vi "Logging Message Loop.vi"(8 "error in (no error)":errorcluster, 10 "DataQueuesAndNotifier":T1, 11 "Message Queues":T2) -> (0 "error out":errorcluster)   [LabVIEW 2019, in "Logging.lvlib"]
doc: "The message loop subVI to handle messages pertaining to logging data."
uses:
  Logging.lvlib
  support/Message Queue/All Message Queues.ctl
  support/Message Queue/Message Cluster.ctl
  Acquisition/DataQueuesAndNotifier.ctl
  Logging State.ctl
  Settings/Settings.ctl
  HardwareAdapter/Support/Hardware Configuration.ctl
  HardwareAdapter/Support/Camera Configuration.ctl
  <vilib>/userdefined/High Color/IMAQdx.ctl
  Logging Configuration.ctl
  controls/UI Configuration.ctl
  controls/CallBack Refs.ctl
  support/Message Queue/Enqueue Message (Single).vi
  <vilib>/Utility/error.llb/Error Cluster From Error Code.vi
  D:/SDK/PMQI-LabViewSamples/Examples/Dependencies/PVCamNET.dll
  E:/DevHardSoftware/MMicroscopy/HardwareAdapter/Lasers/Dependencies/Oxxius_Boxx.dll
  HardwareAdapter/Lasers/Dependencies/Oxxius_Boxx.dll
  <vilib>/ErrorRing/Error Ring.xnode
  support/Message Queue/Message Queue.lvlib
  Settings/Settings.lvlib
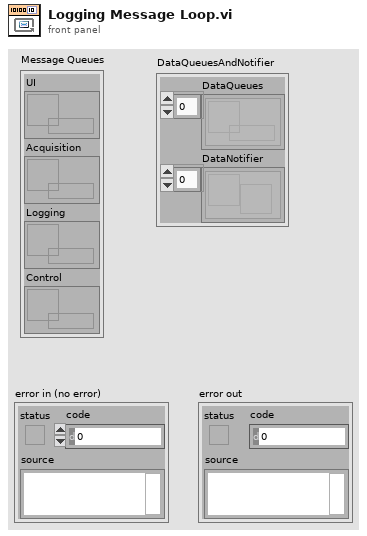
[diagram p1: front panel]
types:
  T1 = typedef "DataQueuesAndNotifier.ctl" = cluster{"DataQueues":refnum<queue>[], "DataNotifier":refnum<notifier>[]}
  T2 = typedef "Message Queue.lvlib/All Message Queues.ctl" = cluster{"UI":refnum<queue>, "Acquisition":refnum<queue>, "Logging":refnum<queue>, "Control":refnum<queue>}
  T3 = typedef "Logging.lvlib/Logging State.ctl" = enum16{"Idle", "Logging"}
  T4 = typedef "Settings.lvlib/Settings.ctl" = cluster{"Hardware Configuration":T5, "Logging Configuration":T8, "HardWare Status":cluster{"CameraAndStages":T9, "Lasers":cluster{"IsConnected":cluster{"405":bool, "488":bool, "532":bool, "561":bool, "647":bool, "785":bool}, "IsOpened":cluster{"405":bool, "488":bool, "532":bool, "561":bool, "647":bool, "785":bool}}}, "CallBack Ref":T10}
  T5 = typedef "Hardware Configuration.ctl" = cluster{"Camera Configuration":T6, "SimpleCamera Configuration":cluster{"Resource":cluster{"Session Out":T7}}, "Stages Configuration":cluster{"Resource":cluster{"NanoStage Ref":i32, "MicroStage Ref":i32, "TirfLock Ref":i32}, "SettingValues":cluster{"NanoState":cluster{"Time":dbl, "X":dbl, "Y":dbl, "Z":dbl}, "MicroState":cluster{"Time 2":dbl, "Z":dbl}, "TirfLock":cluster{"Time":dbl, "X":dbl, "Y":dbl, "Sum":dbl, "Calbrate":dbl, "LockedTarget":dbl, "Kp":dbl, "Ki":dbl, "Avg":dbl}}}, "Lasers Configuration":cluster{"SettingValues":cluster{"405 Power":sgl, "488 Power":sgl, "532 Power":sgl, "561 Power":sgl, "647 Power":sgl, "785 Power":sgl}, "Resource":cluster{"Library Ref":refnum<k24>, "Lasers Ref":cluster{"405 Ref":refnum<k24>, "488 Ref":refnum<k24>, "532 Ref":refnum<k24>, "561 Ref":refnum<k24>, "647 Ref":refnum<k24>, "785 Ref":refnum<k24>}}}}
  T6 = typedef "Camera Configuration.ctl" = cluster{"Resource":cluster{"CameraRef":refnum<k24>, "LibraryRef":refnum<k24>}, "Setting":cluster{"Expouse":dbl, "Frames":dbl, "FrameRate":dbl}}
  T7 = typedef "IMAQdx.ctl" = refnum<k21>
  T8 = typedef "Logging.lvlib/Logging Configuration.ctl" = cluster{"Log File Base Path":path, "FilePrefix":string, "TiffFileFullPath":path, "HardWareInfoFileFullPath":path, "NoteFileFullPath":path}
  T9 = typedef "UI Configuration.ctl" = cluster{"Camera":bool, "NanoStage":bool, "MicroStage":bool, "TIRFLock":bool}
  T10 = typedef "CallBack Refs.ctl" = cluster{"event callback refnum":refnum<k27>, "event callback refnum 2":refnum<k27>, "event callback refnum 3":refnum<k27>, "event callback refnum 4":refnum<k27>}
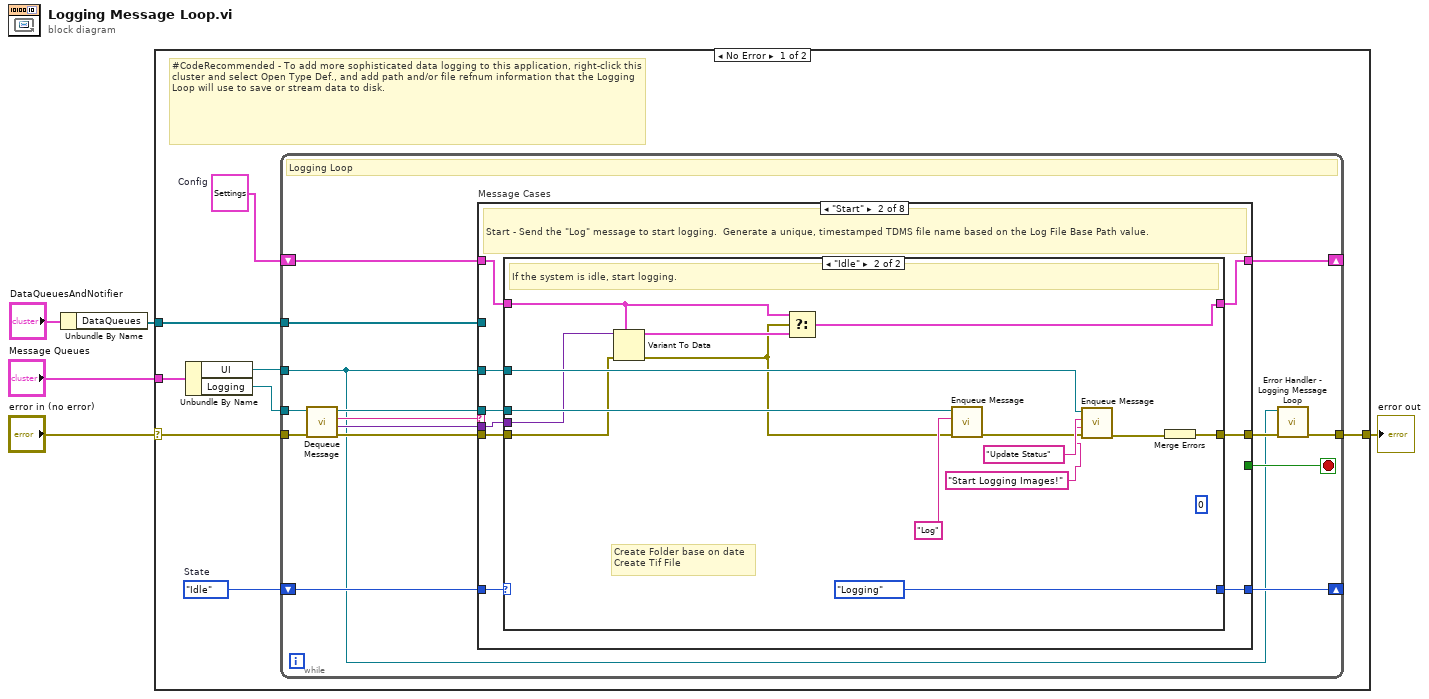
[diagram p0: block diagram]
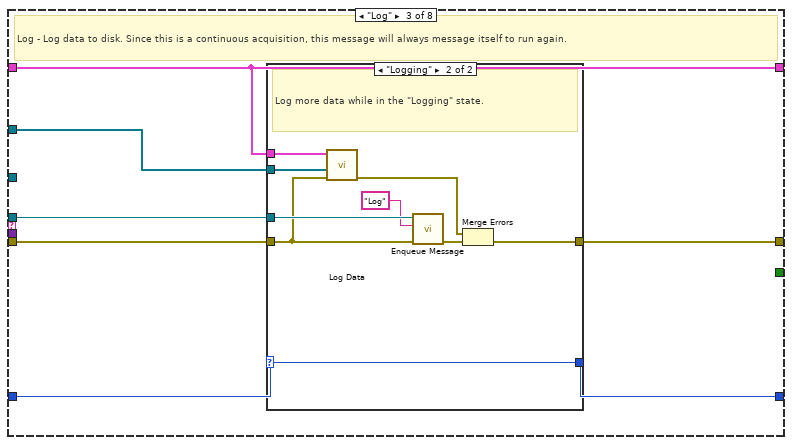
[diagram p4: hidden frame]
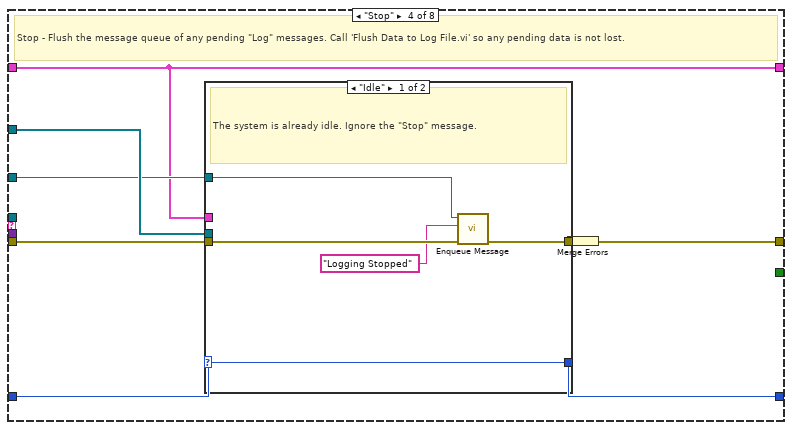
[diagram p6: hidden frame]
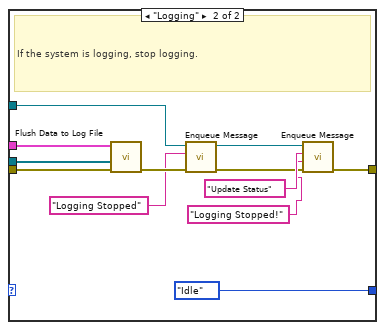
[diagram p7: hidden frame]
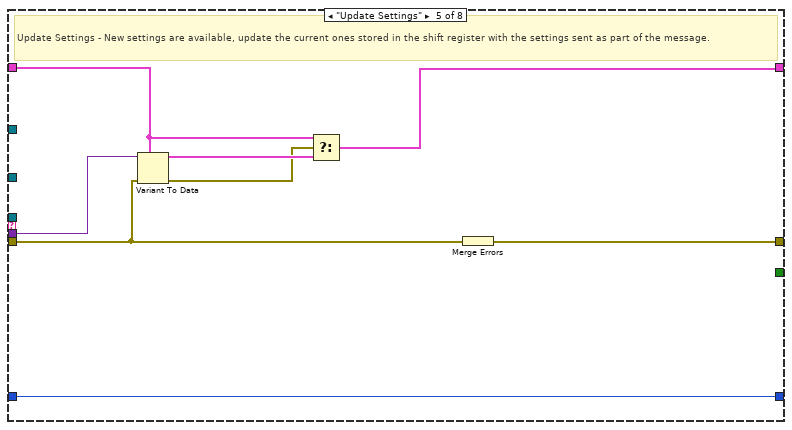
[diagram p8: hidden frame]
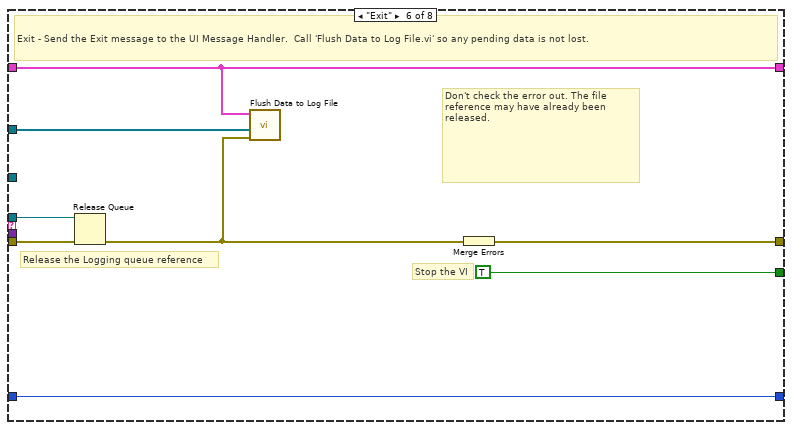
[diagram p9: hidden frame]
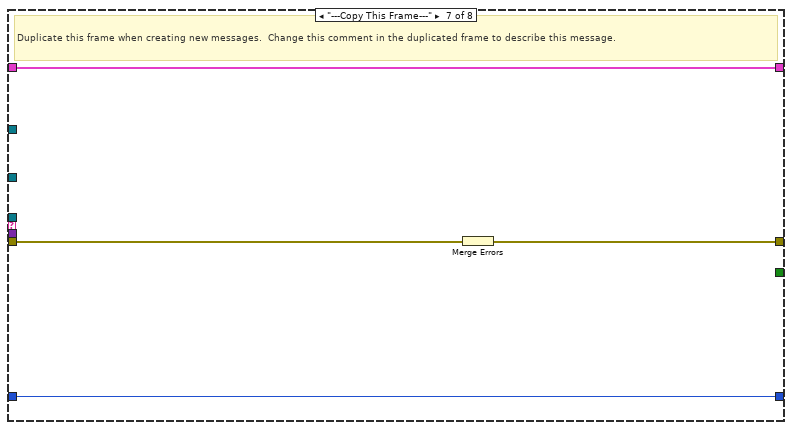
[diagram p10: hidden frame]
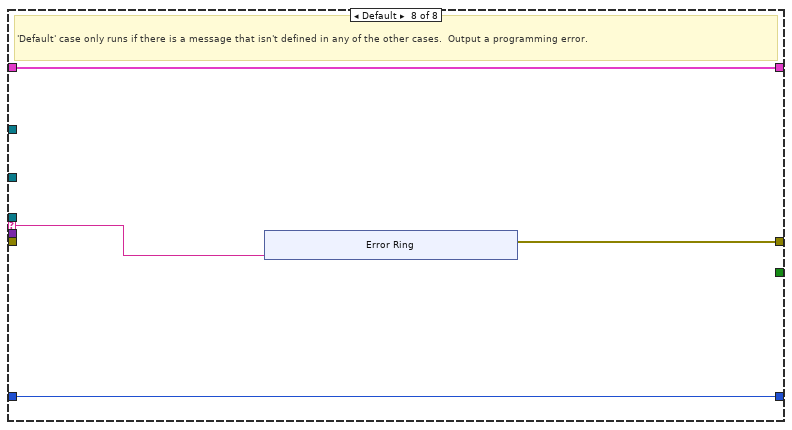
[diagram p11: hidden frame]
diagram:
  n1 = Unbundle By Name("DataQueuesAndNotifier") -> ("DataQueues"=w1:refnum<queue>[])
  n2 = case shown="No Error" "error in (no error)" {
    selector: "error in (no error)" -> [w10 w133]
    tunnel: "Message Queues" -> [w13 _]
    tunnel: [w11 w133] -> w4
    tunnel: w1 -> [w9 _]
    frame No Error {
      w6 = T4 {"Hardware Configuration"={"Camera Configuration"={"Resource"={"CameraRef"=refnum, "LibraryRef"=refnum}, "Setting"={"Expouse"=0.0, "Frames"=0.0, "FrameRate"=0.0}}, "SimpleCamera Configuration"={"Resource"={"Session Out"=""}}, "Stages Configuration"={"Resource"={"NanoStage Ref"=0, "MicroStage Ref"=0, "TirfLock Ref"=0}, "SettingValues"={"NanoState"={"Time"=0.0, "X"=0.0, "Y"=0.0, "Z"=0.0}, "MicroState"={"Time 2"=0.0, "Z"=0.0}, "TirfLock"={"Time"=0.0, "X"=0.0, "Y"=0.0, "Sum"=0.0, "Calbrate"=0.0, "LockedTarget"=0.0, "Kp"=0.0, "Ki"=0.0, "Avg"=0.0}}}, "Lasers Configuration"={"SettingValues"={"405 Power"=0.0, "488 Power"=0.0, "532 Power"=0.0, "561 Power"=0.0, "647 Power"=0.0, "785 Power"=0.0}, "Resource"={"Library Ref"=refnum, "Lasers Ref"={"405 Ref"=refnum, "488 Ref"=refnum, "532 Ref"=refnum, "561 Ref"=refnum, "647 Ref"=refnum, "785 Ref"=refnum}}}}, "Logging Configuration"={"Log File Base Path"=path "", "FilePrefix"="", "TiffFileFullPath"=path "", "HardWareInfoFileFullPath"=path "", "NoteFileFullPath"=path ""}, "HardWare Status"={"CameraAndStages"={"Camera"=FALSE, "NanoStage"=FALSE, "MicroStage"=FALSE, "TIRFLock"=FALSE}, "Lasers"={"IsConnected"={"405"=FALSE, "488"=FALSE, "532"=FALSE, "561"=FALSE, "647"=FALSE, "785"=FALSE}, "IsOpened"={"405"=FALSE, "488"=FALSE, "532"=FALSE, "561"=FALSE, "647"=FALSE, "785"=FALSE}}}, "CallBack Ref"={"event callback refnum"=refnum, "event callback refnum 2"=refnum, "event callback refnum 3"=refnum, "event callback refnum 4"=refnum}}  # Config
      w7 = Logging_State."Idle"  # State
      # "#CodeRecommended - To add more sophisticated data logging to this application, right-click this cluster and select Open Type Def., and add path and/or file refnum information that the Logging Loop will use to save or stream data to disk."
      n3 = Unbundle By Name(w13) -> ("UI"=w8:refnum<queue>, "Logging"=w12:refnum<queue>)
      n4 = while {
        tunnel: w12 -> [w20]
        shift-right: [w27] -> _
        shift-left: w6 -> [w28]
        tunnel: w8 -> [w14]
        tunnel: w9 -> [w19]
        shift-right: [w17] -> _
        shift-left: w7 -> [w18]
        tunnel: w10 -> [w25]
        tunnel: [w16] -> w11
        stop <- w26 stop-if-true
        # "Logging Loop"
        n5 = call "Dequeue Message.vi"("error in (no error)"=w25, "Message Queue"=w20) -> ("error out"=w24:errorcluster, "Message Data"=w22:variant, "Message"=w23:string, "dup Message Queue"=w21:refnum<queue>)  [unwired: 6 in]
        n6 = case "Message Cases" shown="\"Start\"" w23 {
          selector: w23 -> [_ _ _ _ _ _ _ w122]
          tunnel: w21 -> [_ w39 w64 _ _ w114 _ _]
          tunnel: w24 -> [w30 w38 w62 w81 w103 w115 w121 _]
          tunnel: [w30 w40 w65 w84 w109 w116 w119 w123] -> w15
          tunnel: w28 -> [w31 w37 w61 w77 w107 w112 w120 w125]
          tunnel: [w31 w36 w61 w77 w104 w112 w120 w125] -> w27
          tunnel: [_ _ _ _ _ TRUE _ _] -> w26
          tunnel: w22 -> [_ w32 _ _ w108 _ _ _]
          tunnel: w14 -> [_ w33 _ w78 _ _ _ _]
          tunnel: w19 -> [_ _ w63 w82 _ w110 _ _]
          tunnel: w18 -> [w29 w35 w60 w80 w102 w111 w118 w124]
          tunnel: [w29 w34 w59 w79 w102 w111 w118 w124] -> w17
          frame "Initialize" {
            # "Initialize - gets called when first launched. Currently a no-op."
          }
          frame "Start" {
            # "Start - Send the \"Log\" message to start logging.  Generate a unique, timestamped TDMS file name based on the Log File Base Path value."
            n7 = case shown="\"Idle\"" w35 {
              selector: w35 -> [w42 _]
              tunnel: [w41 w57] -> w40
              tunnel: w39 -> [_ w56]
              tunnel: w38 -> [w41 w45]
              tunnel: w37 -> [w43 w47]
              tunnel: [w43 w46] -> w36
              tunnel: [w42 Logging_State."Logging" ("State")] -> w34
              tunnel: w33 -> [_ w50]
              tunnel: w32 -> [_ w48]
              frame "Logging" {
                # "The system is already logging. Ignore the \"Start\" message."
              }
              frame "Idle" {
                (unwired) 0 ("CurrentCaptureFrame")
                # "Create Folder base on date\nCreate Tif File"
                # "If the system is idle, start logging."
                n8 = Variant To Data(error in=w45, type=w47, Variant=w48) -> (data=w49:T4, error out=w44:errorcluster)
                n9 = Select(t=w47, s=w44, f=w49) -> (s? t:f=w46:T4)
                n10 = call-poly "Enqueue Message.vi"("error in (no error)"=w44, "Message"="Log", "Message Queue"=w56) -> ("error out"=w52:errorcluster)  [unwired: 7 in, 1 out]
                n11 = call-poly "Enqueue Message.vi"("error in (no error)"=w52, "Message Data"="Start Logging Images!" ("Message"), "Message"="Update Status", "Message Queue"=w50) -> ("error out"=w51:errorcluster)  [unwired: 6 in, 1 out]
                n12 = Merge Errors(w51) -> (w57:errorcluster)
              }
            }
          }
          frame "Log" {
            # "Log - Log data to disk. Since this is a continuous acquisition, this message will always message itself to run again."
            n13 = case shown="\"Logging\"" w60 {
              selector: w60 -> [w67 w70]
              tunnel: [w66 w76] -> w65
              tunnel: w64 -> [_ w74]
              tunnel: w63 -> [_ w68]
              tunnel: w62 -> [w66 w69]
              tunnel: w61 -> [_ w71]
              tunnel: [w67 w70] -> w59
              frame "Idle" {
                # "Ignore \"Log\" messages when the logging is idle."
              }
              frame "Logging" {
                # "Log more data while in the \"Logging\" state."
                n14 = call "Log Data.vi"("error in (no error)"=w69, "DataQueues"=w68, "Config"=w71) -> ("error out"=w73:errorcluster)  [unwired: 8 in]
                n15 = call-poly "Enqueue Message.vi"("error in (no error)"=w69, "Message"="Log", "Message Queue"=w74) -> ("error out"=w75:errorcluster)  [unwired: 7 in, 1 out]
                n16 = Merge Errors(w73, w75) -> (w76:errorcluster)
              }
            }
          }
          frame "Stop" {
            # "Stop - Flush the message queue of any pending \"Log\" messages. Call 'Flush Data to Log File.vi' so any pending data is not lost."
            n17 = case shown="\"Idle\"" w80 {
              selector: w80 -> [w89 _]
              tunnel: [w87 w91] -> w83
              tunnel: w82 -> [_ w95]
              tunnel: w77 -> [_ w100]
              tunnel: w81 -> [w88 w99]
              tunnel: [w89 Logging_State."Idle" ("State")] -> w79
              tunnel: w78 -> [w85 w97]
              frame "Idle" {
                # "The system is already idle. Ignore the \"Stop\" message."
                n18 = call-poly "Enqueue Message.vi"("error in (no error)"=w88, "Message"="Logging Stopped", "Message Queue"=w85) -> ("error out"=w87:errorcluster)  [unwired: 7 in, 1 out]
              }
              frame "Logging" {
                # "If the system is logging, stop logging."
                n19 = call "Flush Data to Log File.vi"("error in (no error)"=w99, "DataQueues"=w95, "Config"=w100) -> ("error out"=w101:errorcluster)  [unwired: 8 in]
                n20 = call-poly "Enqueue Message.vi"("error in (no error)"=w101, "Message"="Logging Stopped", "Message Queue"=w97) -> ("error out"=w92:errorcluster, "dup Message Queue"=w90:refnum<queue>)  [unwired: 7 in]
                n21 = call-poly "Enqueue Message.vi"("error in (no error)"=w92, "Message Data"="Logging Stopped!" ("Message"), "Message"="Update Status", "Message Queue"=w90) -> ("error out"=w91:errorcluster)  [unwired: 6 in, 1 out]
              }
            }
            n22 = Merge Errors(w83) -> (w84:errorcluster)
          }
          frame "Update Settings" {
            # "Update Settings - New settings are available, update the current ones stored in the shift register with the settings sent as part of the message."
            n23 = Variant To Data(error in=w103, type=w107, Variant=w108) -> (data=w106:T4, error out=w105:errorcluster)
            n24 = Select(t=w107, s=w105, f=w106) -> (s? t:f=w104:T4)
            n25 = Merge Errors(w103) -> (w109:errorcluster)
          }
          frame "Exit" {
            # "Don't check the error out. The file reference may have already been released."
            # "Release the Logging queue reference"
            # "Stop the VI"
            # "Exit - Send the Exit message to the UI Message Handler.  Call 'Flush Data to Log File.vi' so any pending data is not lost."
            n26 = Release Queue(queue=w114, error in (no error)=w115) -> (error out=w113:errorcluster)  [unwired: 1 in, 2 out]
            n27 = call "Flush Data to Log File.vi"("error in (no error)"=w113, "DataQueues"=w110, "Config"=w112) -> ()  [unwired: 8 in, 1 out]
            n28 = Merge Errors(w113) -> (w116:errorcluster)
          }
          frame "---Copy This Frame---" {
            # "Duplicate this frame when creating new messages.  Change this comment in the duplicated frame to describe this message."
            n29 = Merge Errors(w121) -> (w119:errorcluster)
          }
          frame Default {
            # "'Default' case only runs if there is a message that isn't defined in any of the other cases.  Output a programming error."
            n30 = xnode "Error Ring"("parameter 0"=w122) -> ("error out"=w123:errorcluster)
          }
        }
        n31 = call "Error Handler - Logging Message Loop.vi"("error in (no error)"=w15, "Message Queue"=w14) -> ("dup error in"=w16:errorcluster)  [unwired: 8 in, 1 out]
      }
    }
    frame Error {
    }
  }
  "error out" <- w4
